vi "Rate_Set_Sub.vi"(6 "NewVal":T1 format="%#_4g", 7 "VISA resource name":refnum<visa-resource-name>, 8 "Numeric":i32, 9 "Ring Refnum in":refnum<vi>, 11 "Ring in":refnum<vi>) -> (3 "dup VISA Session":refnum<visa-resource-name>)   [LabVIEW 2021]
uses:
  LS336SetRate.ctl
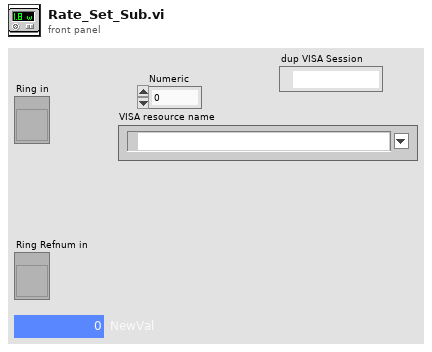
[diagram p1: front panel]
types:
  T1 = typedef "LS336SetRate.ctl" = dbl
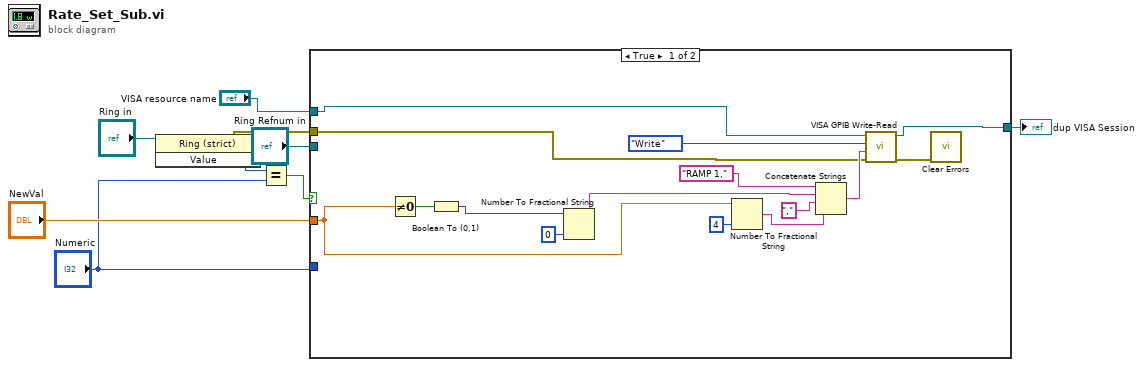
[diagram p0: block diagram]
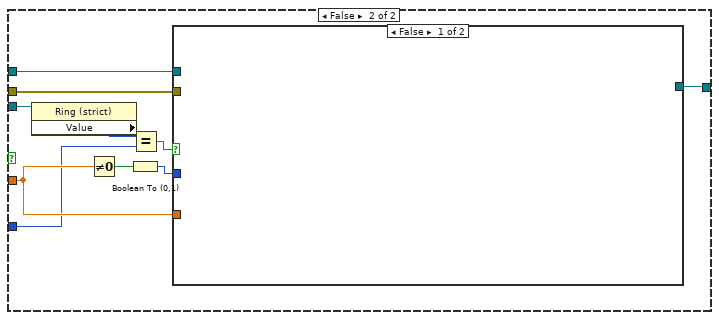
[diagram p2: hidden frame]
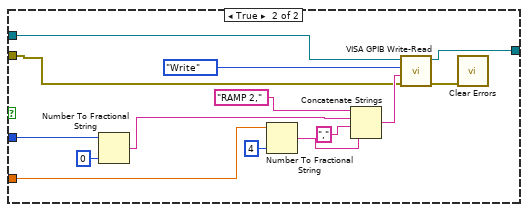
[diagram p3: hidden frame]
diagram:
  n1 = property on="Property Node" class="Ring (strict)"(reference="Ring in") -> (error out=w9:errorcluster, "Value"=w6:u16)  [unwired: 1 in, 1 out]
  n2 = Equal?(x=w6, y="Numeric") -> (x = y?=w7:bool)
  n3 = case shown="True" w7 {
    tunnel: "NewVal" -> [w17 w32]
    tunnel: w9 -> [w11 w34]
    tunnel: "Ring Refnum in" -> [_ w28]
    tunnel: "Numeric" -> [_ w27]
    tunnel: [w12 w26] -> w2
    tunnel: "VISA resource name" -> [w10 w25]
    frame True {
      n4 = Not Equal To 0?(x=w17) -> (x != 0?=w18:bool)
      n5 = Boolean To (0,1)(Boolean=w18) -> (0, 1=w16:i16)
      n6 = Number To Fractional String(number=w16, precision (6)=i16 0) -> (F-format string=w14:string)  [unwired: 2 in]
      n7 = Number To Fractional String(number=w17, precision (6)=i16 4) -> (F-format string=w19:string)  [unwired: 2 in]
      n8 = Concatenate Strings("RAMP 1," ("String to Write"), w14, ",", w19) -> (w21:string)
      n9 = call "VISA GPIB Write-Read.vi"("error in (no error)"=w11, "Command"=w21, "Action"=enum16{"Write", "Read", "Write & Read"}."Write", "VISA resource name"=w10) -> ("error out"=w13:errorcluster, "dup VISA Session"=w12:refnum<visa-resource-name>)  [unwired: 4 in, 2 out]
      n10 = call <vilib>:"Clear Errors.vi"("error in (no error)"=w13) -> ()  [unwired: 5 in, 2 out]
    }
    frame False {
      n11 = property on="Property Node" class="Ring (strict)"(reference=w28) -> ("Value"=w30:u16)  [unwired: 1 in, 2 out]
      n12 = Not Equal To 0?(x=w32) -> (x != 0?=w33:bool)
      n13 = Boolean To (0,1)(Boolean=w33) -> (0, 1=w31:i16)
      n14 = Equal?(x=w30, y=w27) -> (x = y?=w29:bool)
      n15 = case shown="False" w29 {
        tunnel: w34 -> [_ w36]
        tunnel: w32 -> [_ w42]
        tunnel: w31 -> [_ w41]
        tunnel: [_ w37] -> w26
        tunnel: w25 -> [_ w35]
        frame False {
        }
        frame True {
          n16 = Number To Fractional String(number=w41, precision (6)=i16 0) -> (F-format string=w39:string)  [unwired: 2 in]
          n17 = Number To Fractional String(number=w42, precision (6)=i16 4) -> (F-format string=w43:string)  [unwired: 2 in]
          n18 = Concatenate Strings("RAMP 2," ("String to Write"), w39, ",", w43) -> (w45:string)
          n19 = call "VISA GPIB Write-Read.vi"("error in (no error)"=w36, "Command"=w45, "Action"=enum16{"Write", "Read", "Write & Read"}."Write", "VISA resource name"=w35) -> ("error out"=w38:errorcluster, "dup VISA Session"=w37:refnum<visa-resource-name>)  [unwired: 4 in, 2 out]
          n20 = call <vilib>:"Clear Errors.vi"("error in (no error)"=w38) -> ()  [unwired: 5 in, 2 out]
        }
      }
    }
  }
  "dup VISA Session" <- w2
